vi "AMC Local Process Example1.vi"() -> ()   [LabVIEW 2017]
panel:
  out "Process":bool
  in  "OK to Process 2":bool
  out "Status":string
  in  "OK":bool
  in  "Exit":bool
  in  "State Variables":cluster{"CurrentFile":path}
  # "Proccess1"
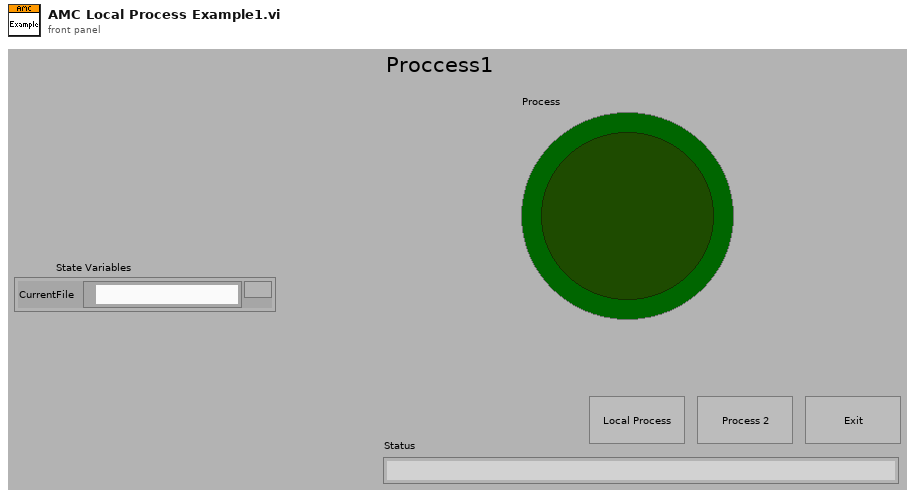
[diagram p1: front panel]
types:
  T1 = typedef "amc_Message Queue.ctl" = refnum<queue>
  T2 = typedef "amc_Message.ctl" = cluster{"Name":string, "Value":string, "Attributes":T3, "Receiver Host":string, "Receiver Process":string, "Source Host":string, "Source Process":string, "Priority Message":bool, "Acknowledge Message":bool}
  T3 = typedef "Tools_KeyedArray KeyedArray.ctl" = cluster{"keys":string[], "values":string[]}
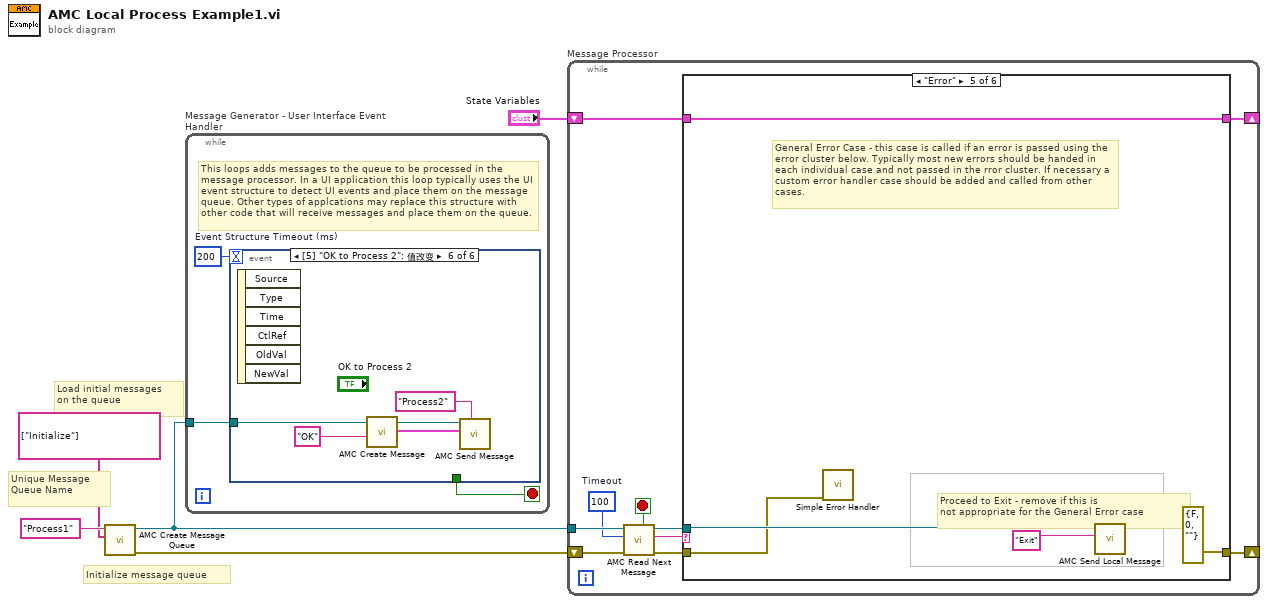
[diagram p0: block diagram]
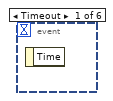
[diagram p2: hidden frame]
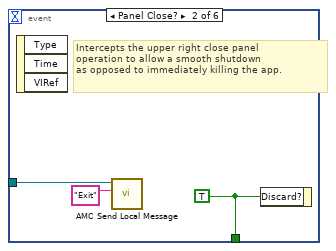
[diagram p3: hidden frame]
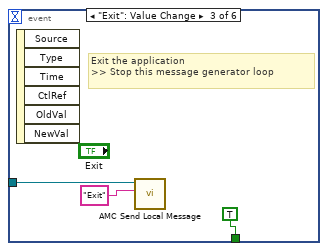
[diagram p4: hidden frame]
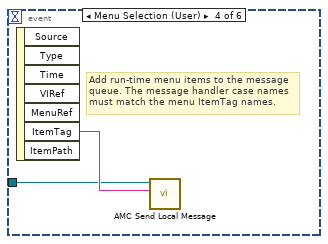
[diagram p5: hidden frame]
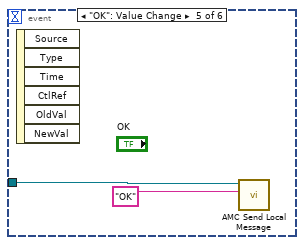
[diagram p6: hidden frame]
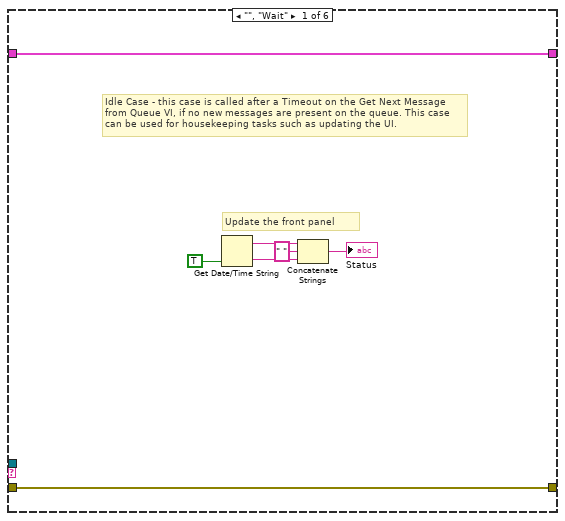
[diagram p7: hidden frame]
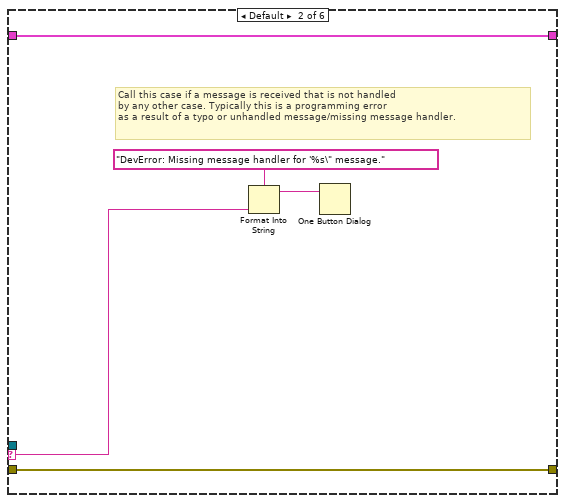
[diagram p8: hidden frame]
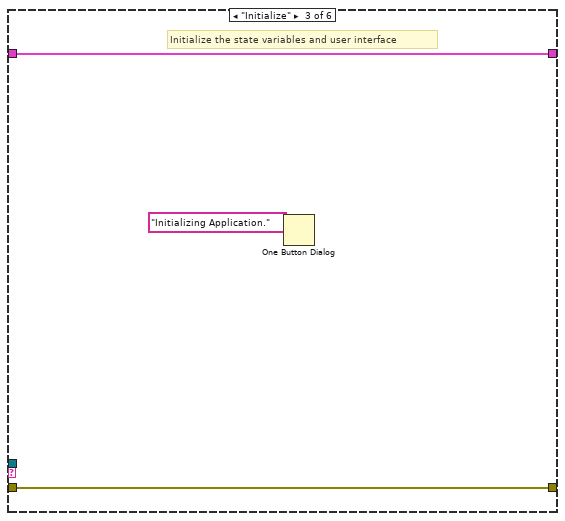
[diagram p9: hidden frame]
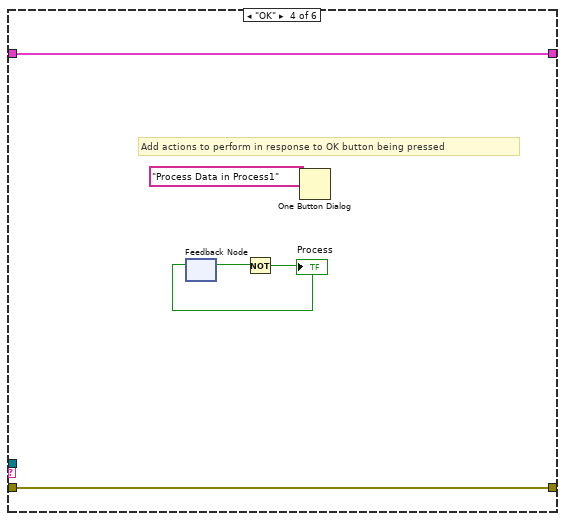
[diagram p10: hidden frame]
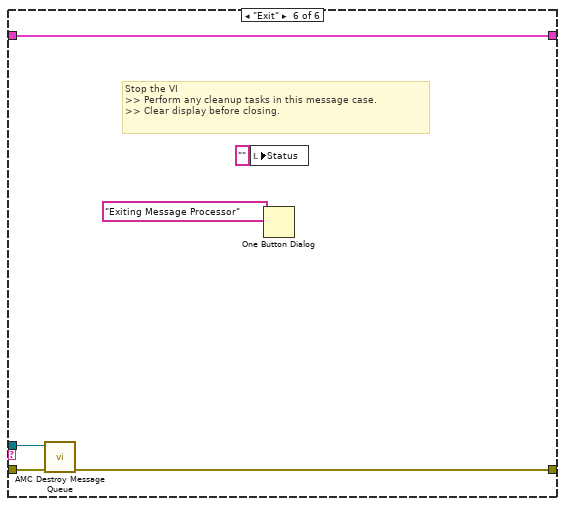
[diagram p11: hidden frame]
diagram:
  # "Initialize message queue"
  # "Unique Message\nQueue Name"
  # "Load initial messages\non the queue"
  n1 = call "AMC Create Message Queue.vi"("Initial Message Names"=string[] ["Initialize"], "Message Queue Name"="Process1" ("Message queue name (unnamed)")) -> ("error out"=w2:errorcluster, "Message Queue out"=w4:T1)  [unwired: 3 in, 5 out]
  n2 = while "Message Generator - User Interface Event Handler" {
    tunnel: w4 -> [w6]
    stop <- w7 stop-if-true
    w8 = 200  # Event Structure Timeout (ms)
    # "This loops adds messages to the queue to be processed in the message processor. In a UI application this loop typically uses the UI event structure to detect UI events and place them on the message queue. Other types of applcations may replace this structure with other code that will receive messages and place them on the queue."
    n3 = event shown="[5] \"OK to Process 2\": 值改变" {
      selector: _ -> [_ _ _ _ _ _]
      dyn-events: _ -> [_ _ _ _ _ _]
      timeout: w8 -> [_ _ _ _ _ _]
      tunnel: [_ w11 TRUE ("Discard?") _ _ _] -> w7
      tunnel: w6 -> [_ w9 w13 w15 w18 w22]
      event Timeout {
        n4 = event-data() -> ()  [unwired: 2 out]
      }
      event Panel Close? {
        w11 = TRUE ("Discard?")
        # "Intercepts the upper right close panel\noperation to allow a smooth shutdown\nas opposed to immediately killing the app."
        n5 = event-data() -> ()  [unwired: 4 out]
        n6 = call "AMC Send Local Message.vi"("Message Name"="Exit", "Message Queue in"=w9) -> ()  [unwired: 4 in, 6 out]
        n7 = event-data("Discard?"=w11) -> ()  [unwired: 1 in, 1 out]
      }
      event "Exit": Value Change {
        # "Exit the application\n>> Stop this message generator loop"
        n8 = event-data() -> ()  [unwired: 7 out]
        n9 = call "AMC Send Local Message.vi"("Message Name"="Exit", "Message Queue in"=w13) -> ()  [unwired: 4 in, 6 out]
      }
      event Menu Selection (User) {
        # "Add run-time menu items to the message\nqueue. The message handler case names must match the menu ItemTag names."
        n10 = event-data() -> ("ItemTag"=w16:string)  [unwired: 7 out]
        n11 = call "AMC Send Local Message.vi"("Message Name"=w16, "Message Queue in"=w15) -> ()  [unwired: 4 in, 6 out]
      }
      event "OK": Value Change {
        n12 = event-data() -> ()  [unwired: 7 out]
        n13 = call "AMC Send Local Message.vi"("Message Name"="OK", "Message Queue in"=w18) -> ()  [unwired: 4 in, 6 out]
      }
      event "OK to Process 2": Value Change {
        n14 = event-data() -> ()  [unwired: 7 out]
        n15 = call "AMC Create Message.vi"("Name"="OK") -> ("Message"=w20:T2)  [unwired: 2 in, 8 out]
        n16 = call "AMC Send Message.vi"("Receiver Process"="Process2" ("process"), "Message"=w20, "Message Queue in"=w22) -> ()  [unwired: 5 in, 4 out]
      }
    }
  }
  n17 = while "Message Processor" {
    shift-left: w2 -> [w27]
    shift-right: [w28] -> _
    tunnel: w4 -> [w26]
    shift-left: "State Variables" -> [w32]
    shift-right: [w31] -> _
    stop <- w25 stop-if-true
    w24 = 100  # Timeout
    n18 = call "AMC Read Next Message.vi"("error in (no error)"=w27, "timeout (1ms)"=w24, "Message Queue in"=w26) -> ("error out"=w29:errorcluster, "Message Name"=w23:string, "Message Queue out"=w30:T1, "Exit Process"=w25:bool)  [unwired: 1 in, 4 out]
    n19 = case shown="\"Error\"" w23 {
      selector: w23 -> [_ w42 _ _ _ _]
      tunnel: [w39 w44 w47 w51 w57 w62] -> w31
      tunnel: w32 -> [w39 w44 w47 w51 w57 w62]
      tunnel: w30 -> [_ _ _ _ w55 w59]
      tunnel: w29 -> [w38 w43 w46 w52 w54 w63]
      tunnel: [w38 w43 w46 w52 errorcluster {"status"=FALSE, "code"=0, "source"=""} ("error out") w61] -> w28
      frame "", "Wait" {
        # "Update the front panel"
        # "Idle Case - this case is called after a Timeout on the Get Next Message from Queue VI, if no new messages are present on the queue. This case can be used for housekeeping tasks such as updating the UI."
        n20 = Get Date/Time String(want seconds? (F)=TRUE) -> (date string=w37:string, time string=w36:string)  [unwired: 2 out]
        n21 = Concatenate Strings(w37, " " ("string"), w36) -> (→"Status":string)
      }
      frame Default {
        # "Call this case if a message is received that is not handled \nby any other case. Typically this is a programming error\nas a result of a typo or unhandled message/missing message handler."
        n22 = Format Into String(format string="DevError: Missing message handler for '%s\" message." ("message"), w42) -> (resulting string=w40:string)  [unwired: 2 in, 1 out]
        n23 = One Button Dialog(message=w40) -> ()  [unwired: 2 out]
      }
      frame "Initialize" {
        # "Initialize the state variables and user interface"
        n24 = One Button Dialog(message="Initializing Application.") -> ()  [unwired: 2 out]
      }
      frame "OK" {
        # "Add actions to perform in response to OK button being pressed"
        n25 = feedback #1() -> (w49:bool)  [unwired: 1 out]
        n26 = Not(x=w49) -> (.not. x?=w48:bool)
        "Process" <- w48
        n27 = feedback-in #1(w48) -> ()
        n28 = One Button Dialog(message="Process Data in Process1") -> ()  [unwired: 2 out]
      }
      frame "Error" {
        # "Proceed to Exit - remove if this is\nnot appropriate for the General Error case"
        # "General Error Case - this case is called if an error is passed using the error cluster below. Typically most new errors should be handed in each individual case and not passed in the rror cluster. If necessary a custom error handler case should be added and called from other cases."
        n29 = call <vilib>:"Simple Error Handler.vi"("error in (no error)"=w54) -> ()  [unwired: 1 in, 8 out]
        n30 = call "AMC Send Local Message.vi"("Message Name"="Exit", "Message Queue in"=w55) -> ()  [unwired: 4 in, 6 out]
      }
      frame "Exit" {
        # "Stop the VI\n>> Perform any cleanup tasks in this message case.\n>> Clear display before closing."
        n31 = call "AMC Destroy Message Queue.vi"("error in (no error)"=w63, "Message Queue in"=w59) -> ("error out"=w61:errorcluster)  [unwired: 9 out]
        n32 = local write "Status"("" ("Status")) -> ()
        n33 = One Button Dialog(message="Exiting Message Processor" ("button name (\"OK\")")) -> ()  [unwired: 2 out]
      }
    }
  }
